vi "Untitled 1.vi"() -> ()   [LabVIEW 2010]
uses:
  <vilib>/picture/picture.llb/Draw True-Color Pixmap.vi
  <userlib>/ImageProcessing/WindowsDriver/LVDS.dll
panel:
  in  "stop 2":bool
  out "new picture":picture
  out "ret":i32
  out "ret 1":i32 format="%x"
  out "ret 3":i32
  out "ret 2":i32 format="%x"
  in  "index":i32
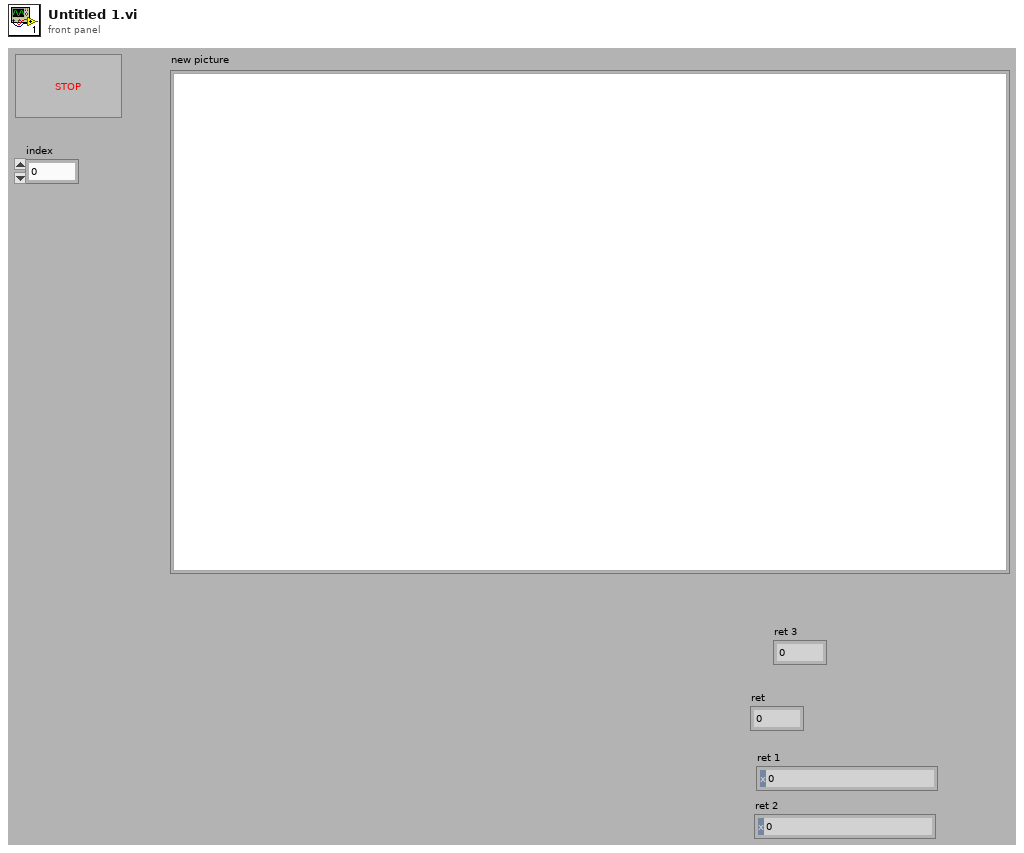
[diagram p1: front panel]
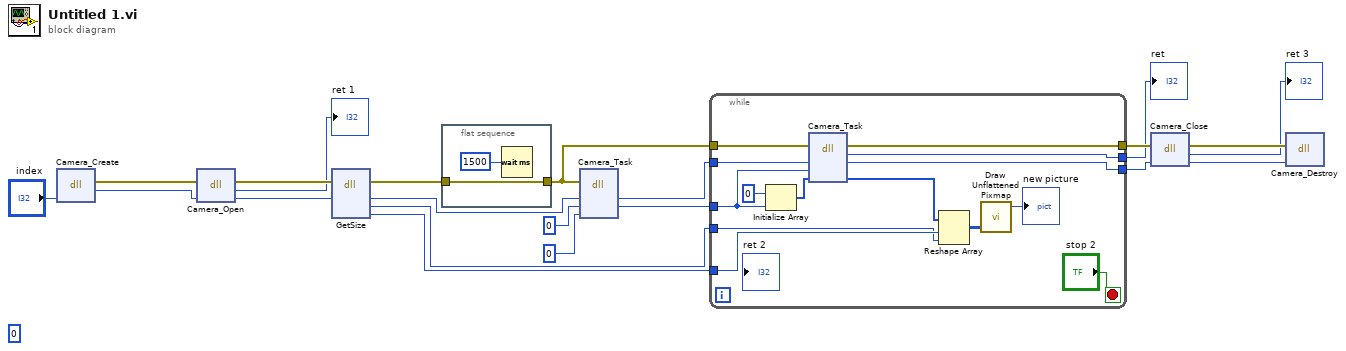
[diagram p0: block diagram]
diagram:
  (unwired) 0 ("element")
  n1 = dll-call lib="C:/Program Files/National Instruments/LabVIEW 2010/user.lib/ImageProcessing/WindowsDriver/LVDS.dll" fn="Camera_Create"("index"="index") -> (error out=w20:errorcluster, "cameraReference"=w19:i64)  [unwired: 4 in, 1 out]
  n2 = dll-call lib="C:/Program Files/National Instruments/LabVIEW 2010/user.lib/ImageProcessing/WindowsDriver/LVDS.dll" fn="Camera_Open"(error in=w20, "cameraReference"=w19) -> (error out=w18:errorcluster, "ret"=→"ret 1":i32, "cameraReference"=w17:i64)  [unwired: 2 in, 1 out]
  n3 = dll-call lib="C:/Program Files/National Instruments/LabVIEW 2010/user.lib/ImageProcessing/WindowsDriver/LVDS.dll" fn="GetSize"(error in=w18, "cameraReference"=w17) -> (error out=w12:errorcluster, "cameraReference"=w3:i64, "width"=w7:i32, "height"=w8:i32)  [unwired: 5 in, 1 out]
  n4 = flat-sequence {
    tunnel: w12 -> [w22]
    tunnel: [w22] -> w4
    frame #0 {
      n5 = Wait (ms)(milliseconds to wait=u32 1500) -> ()  [unwired: 1 out]
    }
  }
  n6 = dll-call lib="C:/Program Files/National Instruments/LabVIEW 2010/user.lib/ImageProcessing/WindowsDriver/LVDS.dll" fn="Camera_Task"(error in=w4, "cameraReference"=w3, "buffersize"=0, "Buffer"=i64 0) -> ("cameraReference"=w2:i64, "buffersize"=w1:i32)  [unwired: 4 in, 2 out]
  n7 = while {
    tunnel: w2 -> [w26]
    tunnel: w4 -> [w25]
    tunnel: [w36] -> w11
    tunnel: [w35] -> w10
    tunnel: [w33] -> w9
    tunnel: w8 -> [w32]
    tunnel: w7 -> [w31]
    tunnel: w1 -> [w24]
    stop <- "stop 2" stop-if-true
    n8 = Initialize Array(0 ("Buffer"), w24) -> (w34:i32[])
    n9 = dll-call lib="C:/Program Files/National Instruments/LabVIEW 2010/user.lib/ImageProcessing/WindowsDriver/LVDS.dll" fn="Camera_Task"(error in=w25, "cameraReference"=w26, "buffersize"=w24, "Buffer"=w34) -> (error out=w35:errorcluster, "ret"=w33:i32, "cameraReference"=w36:i64, "Buffer"=w30:i32[])  [unwired: 3 in, 1 out]
    n10 = Reshape Array(w30, w32, w31) -> (w27:i32[][])
    n11 = call-poly <vilib>:"Draw Unflattened Pixmap.vi"("data (RGB format)"=w27) -> ("new picture"=→"new picture":picture)  [unwired: 8 in]
  }
  "ret" <- w9
  n12 = dll-call lib="C:/Program Files/National Instruments/LabVIEW 2010/user.lib/ImageProcessing/WindowsDriver/LVDS.dll" fn="Camera_Close"(error in=w10, "cameraReference"=w11) -> (error out=w16:errorcluster, "ret"=→"ret 3":i32, "cameraReference"=w15:i64)  [unwired: 2 in, 1 out]
  n13 = dll-call lib="C:/Program Files/National Instruments/LabVIEW 2010/user.lib/ImageProcessing/WindowsDriver/LVDS.dll" fn="Camera_Destroy"(error in=w16, "index"=w15) -> ()  [unwired: 4 in, 2 out]
